vi "Event.vi"() -> ()   [LabVIEW 2019]
panel:
  in  "Boolean":bool
  in  "Numeric":i32
  out "nonevent loop iteration":i32
  out "error out":errorcluster
  out "Numeric Indicator within Event":i32
  out "event loop iteration":i32
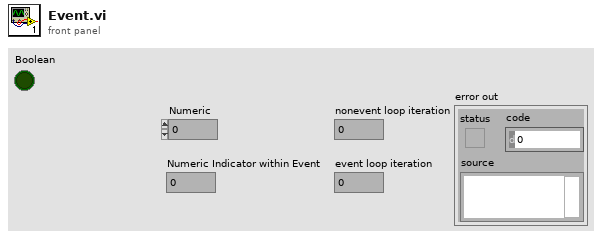
[diagram p1: front panel]
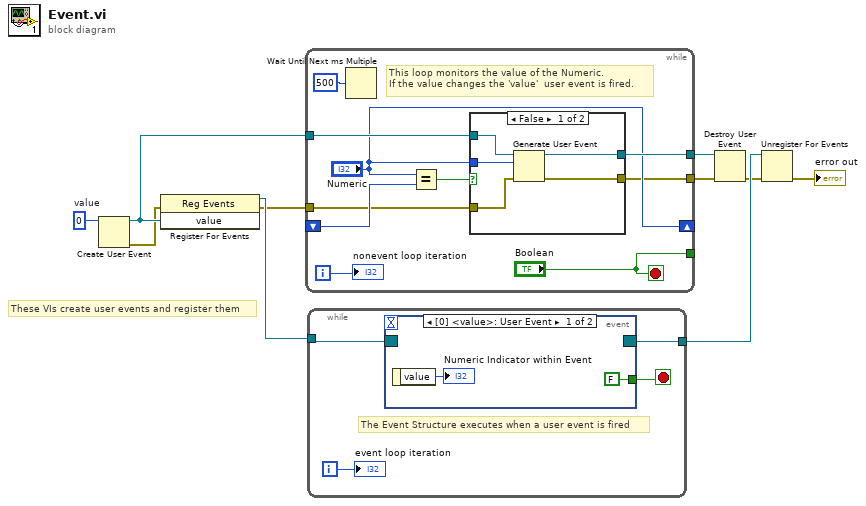
[diagram p0: block diagram]
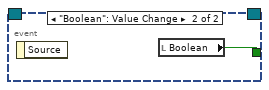
[diagram p3: hidden frame]
diagram:
  w8 = 0  # value
  # "These VIs create user events and register them"
  n1 = Create User Event(user event datatype=w8) -> (user event=w9:refnum<user-event>, error out=w4:errorcluster)  [unwired: 1 in]
  n2 = register-events(error in=w4, w9) -> (reference out=w10:refnum<event-registration>, error out=w3:errorcluster)  [unwired: 1 in]
  n3 = while {
    shift-right: ["Numeric"] -> _
    shift-left: _ -> [w17]
    tunnel: w9 -> [w16]
    tunnel: [w15] -> w1
    tunnel: ["Boolean"] -> _
    tunnel: w3 -> [w13]
    tunnel: [w12] -> w2
    i -> [w18]
    stop <- "Boolean" stop-if-true
    # "This loop monitors the value of the Numeric.\nIf the value changes the 'value'  user event is fired."
    n4 = Wait Until Next ms Multiple(millisecond multiple=u32 500) -> ()  [unwired: 1 out]
    n5 = Equal?(x="Numeric", y=w17) -> (x = y?=w19:bool)
    n6 = case shown="False" w19 {
      tunnel: "Numeric" -> [w24 _]
      tunnel: w16 -> [w25 w27]
      tunnel: [w23 w27] -> w15
      tunnel: w13 -> [w22 w26]
      tunnel: [w21 w26] -> w12
      frame False {
        n7 = Generate User Event(user event=w25, event data cluster=w24, error in=w22) -> (user event out=w23:refnum<user-event>, error out=w21:errorcluster)  [unwired: 1 in]
      }
      frame True {
      }
    }
    "nonevent loop iteration" <- w18
  }
  n8 = while {
    tunnel: w10 -> [w29]
    tunnel: [w28] -> w7
    i -> [w30]
    stop <- w31 stop-if-true
    # "The Event Structure executes when a user event is fired"
    n9 = event shown="[0] <value>: User Event" {
      selector: w29 -> [_ _]
      dyn-events: [_ _] -> w28
      timeout: _ -> [_ _]
      tunnel: [FALSE ("stop") w34] -> w31
      event User Event {
        n10 = event-data() -> ("value"=→"Numeric Indicator within Event":i32)  [unwired: 1 in]
      }
      event "Boolean": Value Change {
        n11 = event-data() -> ()  [unwired: 1 in, 1 out]
        n12 = local read "Boolean"() -> (w34:bool)
      }
    }
    "event loop iteration" <- w30
  }
  n13 = Destroy User Event(user event=w1, error in=w2) -> (error out=w5:errorcluster)
  n14 = Unregister For Events(event registration refnum=w7, error in=w5) -> (error out=→"error out":errorcluster)
